vi "Check if Cluster Control.vi"(0 "typedef cluster":refnum<vi>, 1 "string controls in":string[](array[string]), 2 "controls ref in":refnum<vi>[](array[refnum]), 7 "ctl refnum":refnum<vi>, 9 "vi reference":refnum<vi>, 11 "error in":errorcluster) -> (4 "controls ref out":refnum<vi>[](array[refnum]), 6 "string controls out":string[](array[string]), 15 "error out":errorcluster)   [LabVIEW 2021, in "Converter.lvlib"]
uses:
  Converter.lvlib
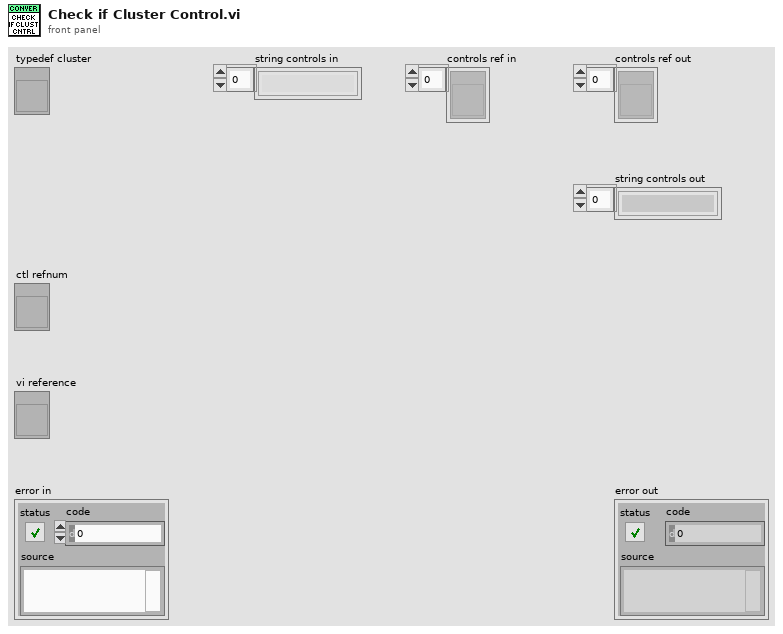
[diagram p1: front panel]
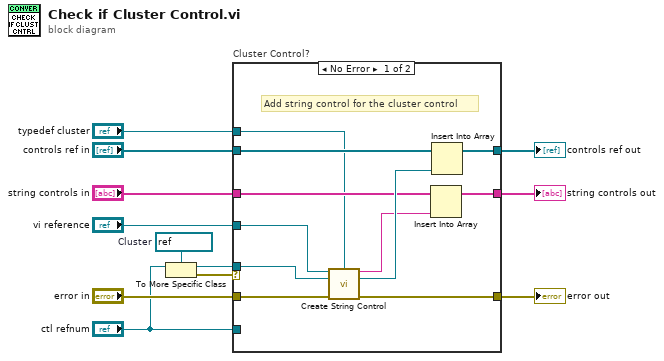
[diagram p0: block diagram]
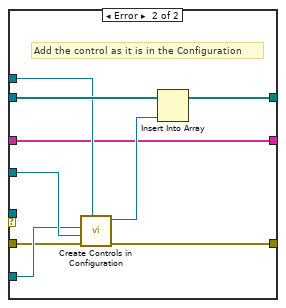
[diagram p2: hidden frame]
diagram:
  w8 = refnum<vi> refnum  # Cluster
  n1 = To More Specific Class(target class=w8, reference="ctl refnum") -> (specific class reference=w10:refnum<vi>, error out=w9:errorcluster)  [unwired: 1 in]
  n2 = case "Cluster Control?" shown="No Error" w9 {
    tunnel: "controls ref in" -> [w19 w32]
    tunnel: [w18 w31] -> w3
    tunnel: "vi reference" -> [w21 w30]
    tunnel: [w22 w28] -> w5
    tunnel: "typedef cluster" -> [w13 w27]
    tunnel: "ctl refnum" -> [_ w26]
    tunnel: "error in" -> [w23 w25]
    tunnel: w10 -> [w20 _]
    tunnel: [w15 w24] -> w11
    tunnel: "string controls in" -> [w16 w24]
    frame No Error {
      # "Add string control for the cluster control"
      n3 = call "Create String Control.vi"("vi refnum"=w21, "typedef cluster"=w13, "clust refnum"=w20, "error in"=w23) -> ("reference string"=w14:string, "string ctl ref"=w17:refnum<vi>, "error out"=w22:errorcluster)  [unwired: 9 in]
      n4 = Insert Into Array(array=w16, new element=w14) -> (w15:string[])  [unwired: 1 in]
      n5 = Insert Into Array(array=w19, new element=w17) -> (w18:refnum<vi>[])  [unwired: 1 in]
    }
    frame Error {
      # "Add the control as it is in the Configuration"
      n6 = call "Create Controls in Configuration.vi"("error in"=w25, "vi refnum"=w30, "ctl refnum"=w26, "cluster ref"=w27) -> ("error out"=w28:errorcluster, "control out"=w29:refnum<vi>)  [unwired: 6 in]
      n7 = Insert Into Array(array=w32, new element=w29) -> (w31:refnum<vi>[])  [unwired: 1 in]
    }
  }
  "string controls out" <- w11
  "error out" <- w5
  "controls ref out" <- w3
